vi "XSens Decode GNSS PVT (SubVI).vi"(5 "DATA In (Hex )":string) -> (0 "Channel Units":string[](array[string])=["NA", "YYYY", "MM", "dd", "hh", "mm", "ss", "NA", "ns", "NA", "NA", "NA", "NA", "DD", "DD", "mm", "mm", "mm", "mm"], 1 "Channel DataTypes":string[](array[string])=["NA", "YYYY", "MM", "dd", "hh", "mm", "ss", "NA", "ns", "NA", "NA", "NA", "NA", "DD", "DD", "mm", "mm", "mm", "mm"], 2 "GPS PVT out":string[](array[string]), 3 "Channel Names":string[](array[string]), 4 "GPS PVT Cluster":T1)   [LabVIEW 2019]
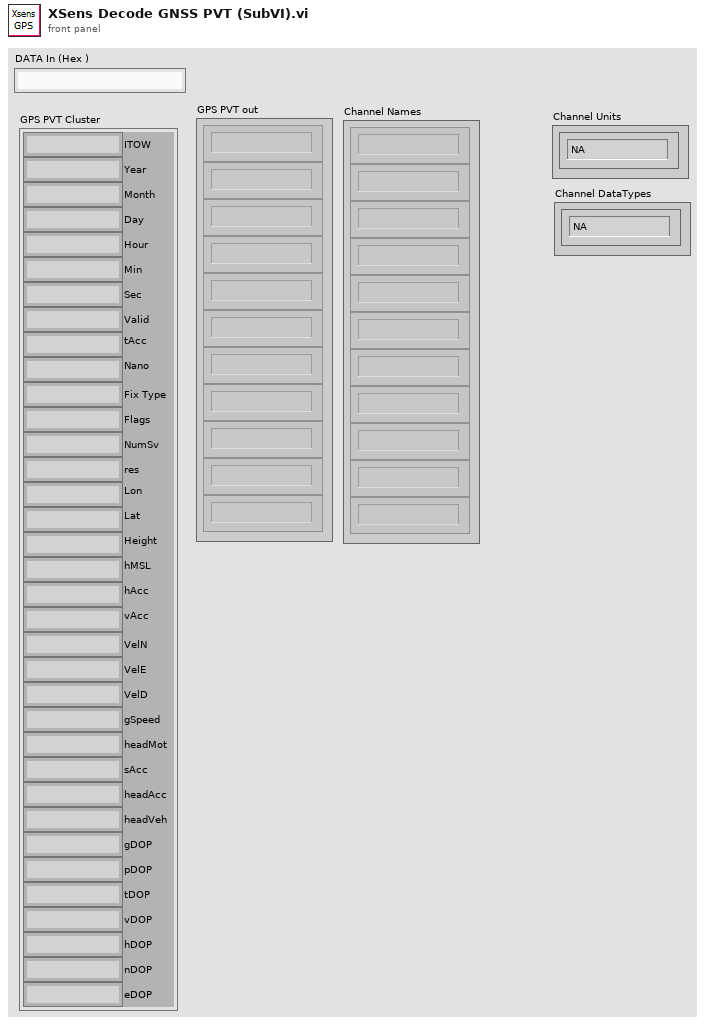
[diagram p1: front panel]
types:
  T1 = cluster{"ITOW":string, "Year":string, "Month":string, "Day":string, "Hour":string, "Min":string, "Sec":string, "Valid":string, "tAcc":string, "Nano":string, "Fix Type":string, "Flags":string, "NumSv":string, "res":string, "Lon":string, "Lat":string, "Height":string, "hMSL":string, "hAcc":string, "vAcc":string, "VelN":string, "VelE":string, "VelD":string, "gSpeed":string, "headMot":string, "sAcc":string, "headAcc":string, "headVeh":string, "gDOP":string, "pDOP":string, "tDOP":string, "vDOP":string, "hDOP":string, "nDOP":string, "eDOP":string}
  T2 = cluster{string, string, string, string, string, string, string, string, string, string, string, string, string, string, string, string, string, string, string, string, string, string, string, string, string, string, string, string, string, string, string, string, string, string, string}
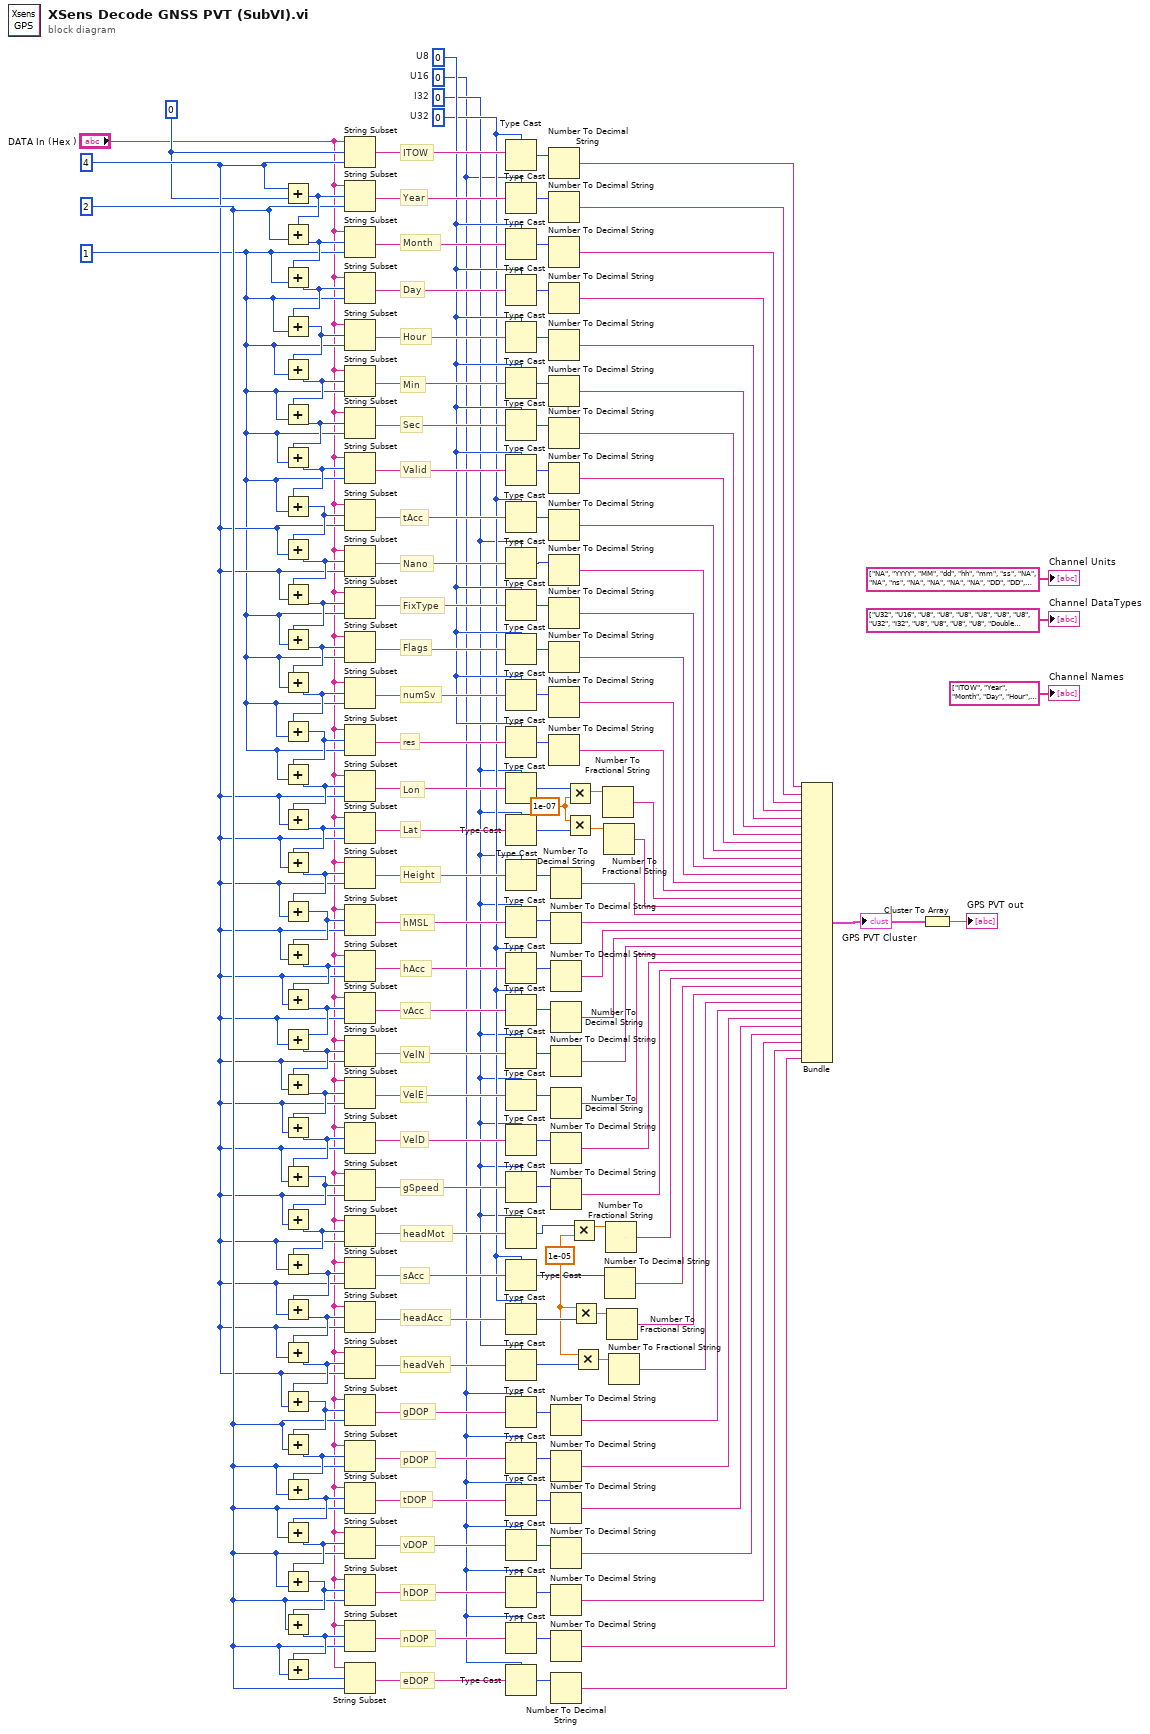
[diagram p0: block diagram]
diagram:
  w77 = 0
  w80 = 1e-05 ("y")
  w84 = 1e-07 ("y")
  w78 = 1 ("length (rest)")
  w90 = 2 ("length (rest)")
  w88 = 0  # I32
  w87 = u16 0  # U16
  w122 = u8 0  # U8
  w89 = u32 0  # U32
  w86 = 4 ("length (rest)")
  # "eDOP"
  # "nDOP"
  # "hDOP"
  # "vDOP"
  # "tDOP"
  # "pDOP"
  # "gDOP"
  # "headVeh"
  # "headAcc"
  # "sAcc"
  # "headMot"
  # "gSpeed"
  # "VelD"
  # "VelE"
  # "VelN"
  # "vAcc"
  # "hAcc"
  # "hMSL"
  # "Height"
  # "Lat"
  # "Lon"
  # "res"
  # "numSv"
  # "Flags"
  # "FixType"
  # "Nano"
  # "tAcc"
  # "Valid"
  # "Sec"
  # "Min"
  # "Hour"
  # "Day"
  # "Month"
  # "Year"
  # "ITOW"
  n1 = Add(x=w86, y=w77) -> (x+y=w149:i32)
  n2 = Add(x=w149, y=w90) -> (x+y=w153:i32)
  n3 = Add(x=w153, y=w78) -> (x+y=w152:i32)
  n4 = Add(x=w152, y=w78) -> (x+y=w151:i32)
  n5 = Add(x=w151, y=w78) -> (x+y=w150:i32)
  n6 = Add(x=w150, y=w78) -> (x+y=w141:i32)
  n7 = Add(x=w141, y=w78) -> (x+y=w144:i32)
  n8 = Add(x=w144, y=w78) -> (x+y=w143:i32)
  n9 = Add(x=w143, y=w86) -> (x+y=w142:i32)
  n10 = Add(x=w142, y=w86) -> (x+y=w123:i32)
  n11 = Add(x=w123, y=w78) -> (x+y=w135:i32)
  n12 = Add(x=w135, y=w78) -> (x+y=w134:i32)
  n13 = Add(x=w134, y=w78) -> (x+y=w133:i32)
  n14 = Add(x=w133, y=w78) -> (x+y=w132:i32)
  n15 = Add(x=w132, y=w86) -> (x+y=w124:i32)
  n16 = Add(x=w124, y=w86) -> (x+y=w127:i32)
  n17 = Add(x=w127, y=w86) -> (x+y=w126:i32)
  n18 = Add(x=w126, y=w86) -> (x+y=w125:i32)
  n19 = Add(x=w125, y=w86) -> (x+y=w91:i32)
  n20 = Add(x=w91, y=w86) -> (x+y=w119:i32)
  n21 = Add(x=w119, y=w86) -> (x+y=w111:i32)
  n22 = Add(x=w111, y=w86) -> (x+y=w114:i32)
  n23 = Add(x=w114, y=w86) -> (x+y=w113:i32)
  n24 = Add(x=w113, y=w86) -> (x+y=w112:i32)
  n25 = Add(x=w112, y=w86) -> (x+y=w92:i32)
  n26 = Add(x=w92, y=w86) -> (x+y=w105:i32)
  n27 = Add(x=w105, y=w86) -> (x+y=w104:i32)
  n28 = Add(x=w104, y=w86) -> (x+y=w103:i32)
  n29 = Add(x=w103, y=w90) -> (x+y=w102:i32)
  n30 = Add(x=w102, y=w90) -> (x+y=w93:i32)
  n31 = Add(x=w93, y=w90) -> (x+y=w96:i32)
  n32 = Add(x=w96, y=w90) -> (x+y=w95:i32)
  n33 = Add(x=w95, y=w90) -> (x+y=w94:i32)
  n34 = Add(x=w94, y=w90) -> (x+y=w97:i32)
  n35 = String Subset(string="DATA In (Hex )", offset (0)=w77, length (rest)=w86) -> (substring=w160:string)
  n36 = String Subset(string="DATA In (Hex )", offset (0)=w149, length (rest)=w90) -> (substring=w159:string)
  n37 = String Subset(string="DATA In (Hex )", offset (0)=w153, length (rest)=w78) -> (substring=w158:string)
  n38 = String Subset(string="DATA In (Hex )", offset (0)=w152, length (rest)=w78) -> (substring=w157:string)
  n39 = String Subset(string="DATA In (Hex )", offset (0)=w151, length (rest)=w78) -> (substring=w156:string)
  n40 = String Subset(string="DATA In (Hex )", offset (0)=w150, length (rest)=w78) -> (substring=w155:string)
  n41 = String Subset(string="DATA In (Hex )", offset (0)=w141, length (rest)=w78) -> (substring=w154:string)
  n42 = String Subset(string="DATA In (Hex )", offset (0)=w144, length (rest)=w78) -> (substring=w148:string)
  n43 = String Subset(string="DATA In (Hex )", offset (0)=w143, length (rest)=w86) -> (substring=w147:string)
  n44 = String Subset(string="DATA In (Hex )", offset (0)=w142, length (rest)=w86) -> (substring=w146:string)
  n45 = String Subset(string="DATA In (Hex )", offset (0)=w123, length (rest)=w78) -> (substring=w145:string)
  n46 = String Subset(string="DATA In (Hex )", offset (0)=w135, length (rest)=w78) -> (substring=w140:string)
  n47 = String Subset(string="DATA In (Hex )", offset (0)=w134, length (rest)=w78) -> (substring=w139:string)
  n48 = String Subset(string="DATA In (Hex )", offset (0)=w133, length (rest)=w78) -> (substring=w138:string)
  n49 = String Subset(string="DATA In (Hex )", offset (0)=w132, length (rest)=w86) -> (substring=w137:string)
  n50 = String Subset(string="DATA In (Hex )", offset (0)=w124, length (rest)=w86) -> (substring=w136:string)
  n51 = String Subset(string="DATA In (Hex )", offset (0)=w127, length (rest)=w86) -> (substring=w131:string)
  n52 = String Subset(string="DATA In (Hex )", offset (0)=w126, length (rest)=w86) -> (substring=w130:string)
  n53 = String Subset(string="DATA In (Hex )", offset (0)=w125, length (rest)=w86) -> (substring=w129:string)
  n54 = String Subset(string="DATA In (Hex )", offset (0)=w91, length (rest)=w86) -> (substring=w128:string)
  n55 = String Subset(string="DATA In (Hex )", offset (0)=w119, length (rest)=w86) -> (substring=w121:string)
  n56 = String Subset(string="DATA In (Hex )", offset (0)=w111, length (rest)=w86) -> (substring=w120:string)
  n57 = String Subset(string="DATA In (Hex )", offset (0)=w114, length (rest)=w86) -> (substring=w118:string)
  n58 = String Subset(string="DATA In (Hex )", offset (0)=w113, length (rest)=w86) -> (substring=w117:string)
  n59 = String Subset(string="DATA In (Hex )", offset (0)=w112, length (rest)=w86) -> (substring=w116:string)
  n60 = String Subset(string="DATA In (Hex )", offset (0)=w92, length (rest)=w86) -> (substring=w115:string)
  n61 = String Subset(string="DATA In (Hex )", offset (0)=w105, length (rest)=w86) -> (substring=w110:string)
  n62 = String Subset(string="DATA In (Hex )", offset (0)=w104, length (rest)=w86) -> (substring=w109:string)
  n63 = String Subset(string="DATA In (Hex )", offset (0)=w103, length (rest)=w90) -> (substring=w108:string)
  n64 = String Subset(string="DATA In (Hex )", offset (0)=w102, length (rest)=w90) -> (substring=w107:string)
  n65 = String Subset(string="DATA In (Hex )", offset (0)=w93, length (rest)=w90) -> (substring=w106:string)
  n66 = String Subset(string="DATA In (Hex )", offset (0)=w96, length (rest)=w90) -> (substring=w101:string)
  n67 = String Subset(string="DATA In (Hex )", offset (0)=w95, length (rest)=w90) -> (substring=w100:string)
  n68 = String Subset(string="DATA In (Hex )", offset (0)=w94, length (rest)=w90) -> (substring=w99:string)
  n69 = String Subset(string="DATA In (Hex )", offset (0)=w97, length (rest)=w90) -> (substring=w98:string)
  n70 = Type Cast(type=w89, x=w160) -> (*(type *) &x=w76:u32)
  n71 = Type Cast(type=w87, x=w159) -> (*(type *) &x=w74:u16)
  n72 = Type Cast(type=w122, x=w158) -> (*(type *) &x=w72:u8)
  n73 = Type Cast(type=w122, x=w157) -> (*(type *) &x=w70:u8)
  n74 = Type Cast(type=w122, x=w156) -> (*(type *) &x=w68:u8)
  n75 = Type Cast(type=w122, x=w155) -> (*(type *) &x=w66:u8)
  n76 = Type Cast(type=w122, x=w154) -> (*(type *) &x=w64:u8)
  n77 = Type Cast(type=w122, x=w148) -> (*(type *) &x=w62:u8)
  n78 = Type Cast(type=w89, x=w147) -> (*(type *) &x=w60:u32)
  n79 = Type Cast(type=w88, x=w146) -> (*(type *) &x=w58:i32)
  n80 = Type Cast(type=w122, x=w145) -> (*(type *) &x=w56:u8)
  n81 = Type Cast(type=w122, x=w140) -> (*(type *) &x=w54:u8)
  n82 = Type Cast(type=w122, x=w139) -> (*(type *) &x=w52:u8)
  n83 = Type Cast(type=w122, x=w138) -> (*(type *) &x=w50:u8)
  n84 = Type Cast(type=w88, x=w137) -> (*(type *) &x=w85:i32)
  n85 = Type Cast(type=w88, x=w136) -> (*(type *) &x=w83:i32)
  n86 = Type Cast(type=w88, x=w131) -> (*(type *) &x=w44:i32)
  n87 = Type Cast(type=w88, x=w130) -> (*(type *) &x=w42:i32)
  n88 = Type Cast(type=w89, x=w129) -> (*(type *) &x=w40:u32)
  n89 = Type Cast(type=w89, x=w128) -> (*(type *) &x=w38:u32)
  n90 = Type Cast(type=w88, x=w121) -> (*(type *) &x=w36:i32)
  n91 = Type Cast(type=w88, x=w120) -> (*(type *) &x=w34:i32)
  n92 = Type Cast(type=w88, x=w118) -> (*(type *) &x=w32:i32)
  n93 = Type Cast(type=w88, x=w117) -> (*(type *) &x=w30:i32)
  n94 = Type Cast(type=w88, x=w116) -> (*(type *) &x=w82:i32)
  n95 = Type Cast(type=w89, x=w115) -> (*(type *) &x=w26:u32)
  n96 = Type Cast(type=w89, x=w110) -> (*(type *) &x=w81:u32)
  n97 = Type Cast(type=w88, x=w109) -> (*(type *) &x=w79:i32)
  n98 = Type Cast(type=w87, x=w108) -> (*(type *) &x=w20:u16)
  n99 = Type Cast(type=w87, x=w107) -> (*(type *) &x=w18:u16)
  n100 = Type Cast(type=w87, x=w106) -> (*(type *) &x=w16:u16)
  n101 = Type Cast(type=w87, x=w101) -> (*(type *) &x=w14:u16)
  n102 = Type Cast(type=w87, x=w100) -> (*(type *) &x=w12:u16)
  n103 = Type Cast(type=w87, x=w99) -> (*(type *) &x=w10:u16)
  n104 = Type Cast(type=w87, x=w98) -> (*(type *) &x=w8:u16)
  n105 = Number To Decimal String(number=w76) -> (decimal integer string=w75:string)  [unwired: 1 in]
  n106 = Number To Decimal String(number=w74) -> (decimal integer string=w73:string)  [unwired: 1 in]
  n107 = Number To Decimal String(number=w72) -> (decimal integer string=w71:string)  [unwired: 1 in]
  n108 = Number To Decimal String(number=w70) -> (decimal integer string=w69:string)  [unwired: 1 in]
  n109 = Number To Decimal String(number=w68) -> (decimal integer string=w67:string)  [unwired: 1 in]
  n110 = Number To Decimal String(number=w66) -> (decimal integer string=w65:string)  [unwired: 1 in]
  n111 = Number To Decimal String(number=w64) -> (decimal integer string=w63:string)  [unwired: 1 in]
  n112 = Number To Decimal String(number=w62) -> (decimal integer string=w61:string)  [unwired: 1 in]
  n113 = Number To Decimal String(number=w60) -> (decimal integer string=w59:string)  [unwired: 1 in]
  n114 = Number To Decimal String(number=w58) -> (decimal integer string=w57:string)  [unwired: 1 in]
  n115 = Number To Decimal String(number=w56) -> (decimal integer string=w55:string)  [unwired: 1 in]
  n116 = Number To Decimal String(number=w54) -> (decimal integer string=w53:string)  [unwired: 1 in]
  n117 = Number To Decimal String(number=w52) -> (decimal integer string=w51:string)  [unwired: 1 in]
  n118 = Number To Decimal String(number=w50) -> (decimal integer string=w49:string)  [unwired: 1 in]
  n119 = Number To Decimal String(number=w44) -> (decimal integer string=w43:string)  [unwired: 1 in]
  n120 = Number To Decimal String(number=w42) -> (decimal integer string=w41:string)  [unwired: 1 in]
  n121 = Number To Decimal String(number=w40) -> (decimal integer string=w39:string)  [unwired: 1 in]
  n122 = Number To Decimal String(number=w38) -> (decimal integer string=w37:string)  [unwired: 1 in]
  n123 = Number To Decimal String(number=w36) -> (decimal integer string=w35:string)  [unwired: 1 in]
  n124 = Number To Decimal String(number=w34) -> (decimal integer string=w33:string)  [unwired: 1 in]
  n125 = Number To Decimal String(number=w32) -> (decimal integer string=w31:string)  [unwired: 1 in]
  n126 = Number To Decimal String(number=w30) -> (decimal integer string=w29:string)  [unwired: 1 in]
  n127 = Number To Decimal String(number=w20) -> (decimal integer string=w19:string)  [unwired: 1 in]
  n128 = Number To Decimal String(number=w18) -> (decimal integer string=w17:string)  [unwired: 1 in]
  n129 = Number To Decimal String(number=w16) -> (decimal integer string=w15:string)  [unwired: 1 in]
  n130 = Number To Decimal String(number=w14) -> (decimal integer string=w13:string)  [unwired: 1 in]
  n131 = Number To Decimal String(number=w12) -> (decimal integer string=w11:string)  [unwired: 1 in]
  n132 = Number To Decimal String(number=w10) -> (decimal integer string=w9:string)  [unwired: 1 in]
  n133 = Number To Decimal String(number=w8) -> (decimal integer string=w7:string)  [unwired: 1 in]
  n134 = Multiply(x=w85, y=w84) -> (x*y=w48:dbl)
  n135 = Multiply(x=w84, y=w83) -> (x*y=w46:dbl)
  n136 = Multiply(x=w82, y=w80) -> (x*y=w28:dbl)
  n137 = Multiply(x=w80, y=w81) -> (x*y=w24:dbl)
  n138 = Multiply(x=w80, y=w79) -> (x*y=w22:dbl)
  n139 = Number To Fractional String(number=w48) -> (F-format string=w47:string)  [unwired: 3 in]
  n140 = Number To Fractional String(number=w46) -> (F-format string=w45:string)  [unwired: 3 in]
  n141 = Number To Decimal String(number=w26) -> (decimal integer string=w25:string)  [unwired: 1 in]
  n142 = Number To Fractional String(number=w28) -> (F-format string=w27:string)  [unwired: 3 in]
  n143 = Number To Fractional String(number=w24) -> (F-format string=w23:string)  [unwired: 3 in]
  n144 = Number To Fractional String(number=w22) -> (F-format string=w21:string)  [unwired: 3 in]
  n145 = Bundle(w75, w73, w71, w69, w67, w65, w63, w61, w59, w57, w55, w53, w51, w49, w47, w45, w43, w41, w39, w37, w35, w33, w31, w29, w27, w25, w23, w21, w19, w17, w15, w13, w11, w9, w7) -> (w3:T2)  [unwired: 1 in]
  "GPS PVT Cluster" <- w3
  n146 = Cluster To Array(cluster=w3) -> (array=→"GPS PVT out":string[])
  "Channel Units" <- string[] ["NA", "YYYY", "MM", "dd", "hh", "mm", "ss", "NA", "NA", "ns", "NA", "NA", "NA", "NA", "DD", "DD", "mm", "mm", "mm", "mm", "mm/s", "mm/s", "mm/s", "mm/s", "deg", "mm/s", "deg", "deg", "NA", "NA", "NA", "NA", "NA", "NA", "NA"] ("Channel Names")
  "Channel Names" <- string[] ["ITOW", "Year", "Month", "Day", "Hour", "Min", "Sec", "Valid", "tAcc", "Nano", "Fix Type", "Flags", "NumSv", "res", "Lon", "Lat", "Height", "hMSL", "hAcc", "vAcc", "VelN", "VelE", "VelD", "gSpeed", "headMot", "sAcc", "headAcc", "headVeh", "gDOP", "pDOP", "tDOP", "vDOP", "hDOP", "nDOP", "eDOP"] ("Channel Names")
  "Channel DataTypes" <- string[] ["U32", "U16", "U8", "U8", "U8", "U8", "U8", "U8", "U32", "I32", "U8", "U8", "U8", "U8", "Double Float", "Double Float", "I32", "I32", "U32", "U32", "I32", "I32", "I32", "I32", "I32", "U32", "U32", "I32", "U16", "U16", "U16", "U16", "U16", "U16", "U16"] ("Channel Names")
